vi "Galvo.vi"() -> ()   [LabVIEW 2018]
panel:
  out "电压1":dbl(graph)
  out "电压2":dbl(graph)
  in  "扫描时间间隔(s)":dbl
  out "光开关":bool
  out "电压2":dbl
  out "电压1":dbl
  out "文件预览":string
  in  "输入转角文件路径：":T1
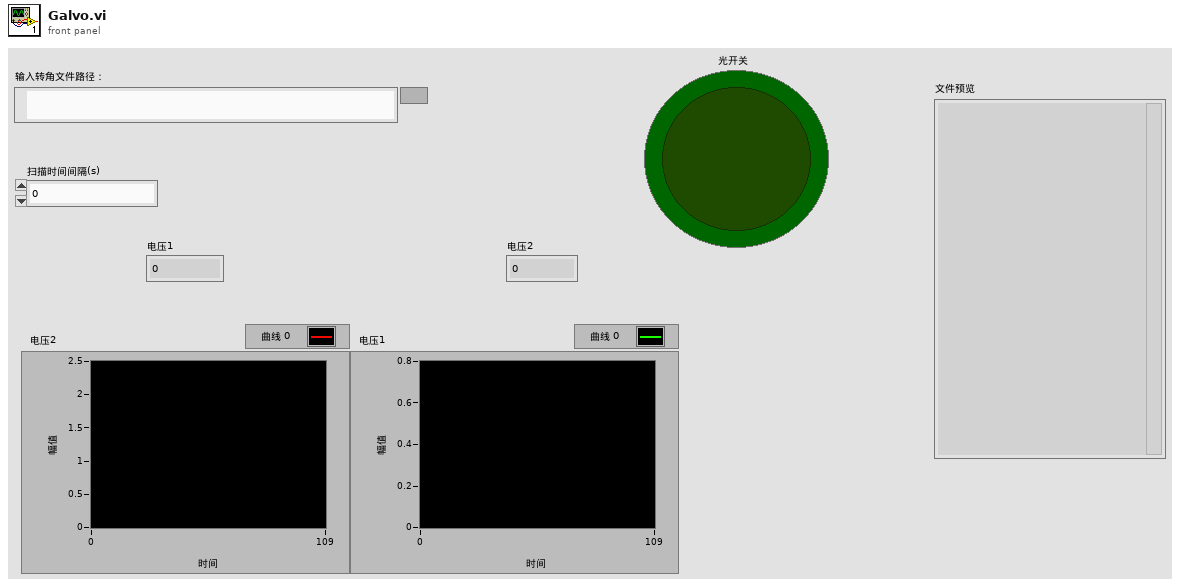
[diagram p1: front panel]
types:
  T1 = typedef "控件 1.ctl" = path
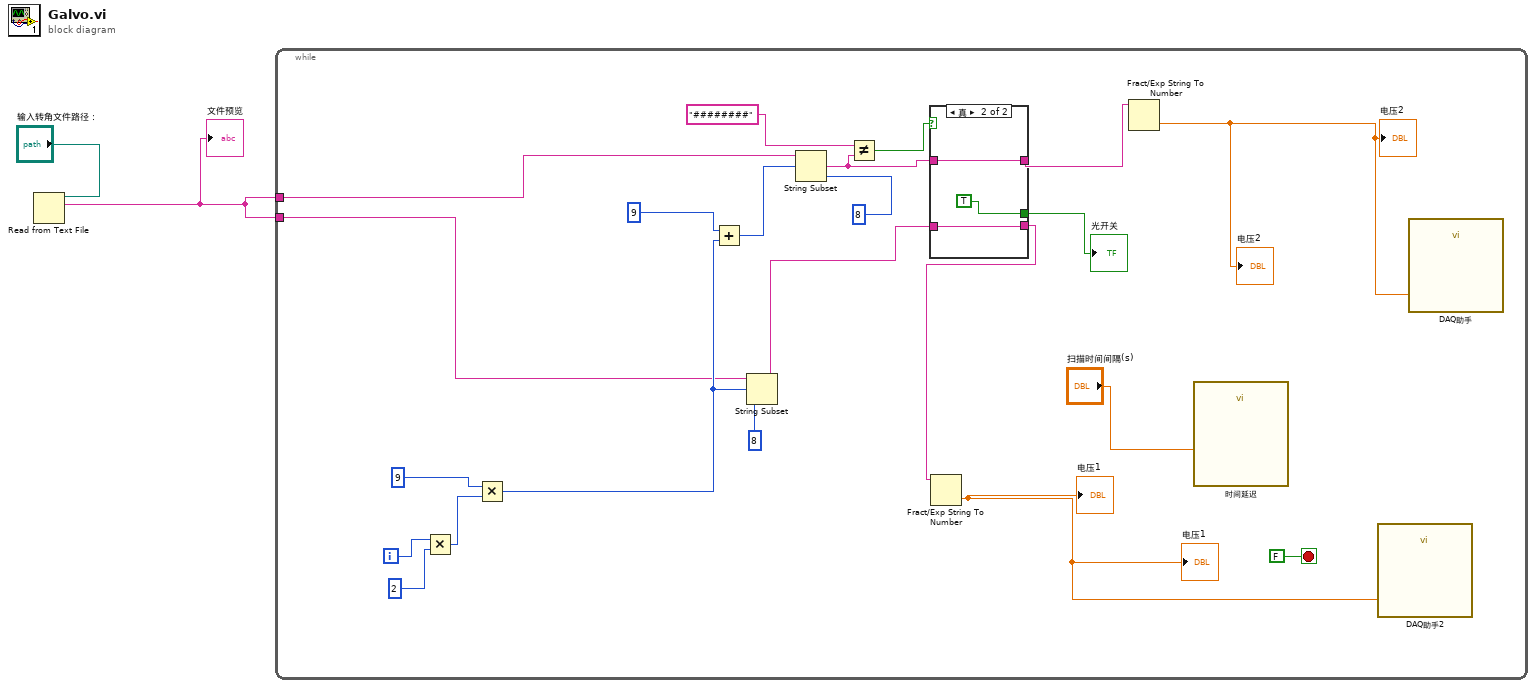
[diagram p0: block diagram]
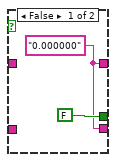
[diagram p2: hidden frame]
diagram:
  n1 = Read from Text File(file (use dialog)="输入转角文件路径：") -> (text=w1:string)  [unwired: 3 in, 3 out]
  "文件预览" <- w1
  n2 = while {
    tunnel: w1 -> [w13]
    tunnel: w1 -> [w14]
    i -> [w16]
    stop <- FALSE stop-if-true
    n3 = Multiply(x=w16, y=2) -> (x*y=w15:i32)
    n4 = Multiply(x=9, y=w15) -> (x*y=w19:i32)
    n5 = Add(x=9, y=w19) -> (x+y=w18:i32)
    n6 = String Subset(string=w13, offset (0)=w19, length (rest)=8) -> (substring=w7:string)
    n7 = String Subset(string=w14, offset (0)=w18, length (rest)=8) -> (substring=w9:string)
    n8 = Not Equal?(x="########", y=w9) -> (x != y?=w8:bool)
    n9 = case shown="真" w8 {
      tunnel: w9 -> [_ w29]
      tunnel: [w25 w29] -> w12
      tunnel: [FALSE TRUE] -> w11
      tunnel: [w25 w27] -> w6
      tunnel: w7 -> [_ w27]
      frame False {
        w25 = "0.000000"
      }
      frame True {
      }
    }
    "光开关" <- w11
    n10 = Fract/Exp String To Number(string=w6) -> (number=w3:dbl)  [unwired: 3 in, 1 out]
    "电压1" <- w3
    "电压1" <- w3
    n11 = Fract/Exp String To Number(string=w12) -> (number=w4:dbl)  [unwired: 3 in, 1 out]
    "电压2" <- w4
    "电压2" <- w4
    n12 = call "时间延迟"("Delay Time (s)"="扫描时间间隔(s)") -> ()  [unwired: 10 in, 1 out]
    n13 = call "DAQ助手2"("data"=w3) -> ()  [unwired: 17 in, 2 out]
    n14 = call "DAQ助手"("data"=w4) -> ()  [unwired: 17 in, 2 out]
  }
